vi "Theme4_Topic2_qn8.vi"(9 "RefPrevious":refnum<vi>, 10 "RefNext":refnum<vi>, 11 "connection reference":T1) -> (2 "AnsIndicator":refnum<vi>[](array[refnum]))   [LabVIEW 2013]
uses:
  why.vi
  Precontrol.vi
  <vilib>/addons/database/Connection.llb/Conn ObjectReference.ctl
  <vilib>/addons/database/NI_Database_API.lvlib
panel:
  out "Why?":string
  out "DInd":bool
  out "CInd":bool
  out "BInd":bool
  out "AInd":bool
  in  "ABCD":enum32{"No Selection", "A", "B", "C", "D"}(radio)
  out "MCQ_Randomized":string[](array[string])
  # "The speed of a wave is affected by _____________________."
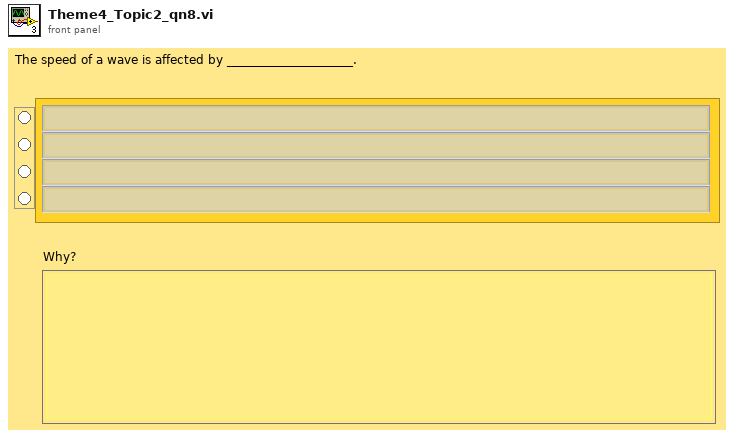
[diagram p1: front panel]
types:
  T1 = typedef "NI_Database_API.lvlib/Conn ObjectReference.ctl" = refnum<k1>
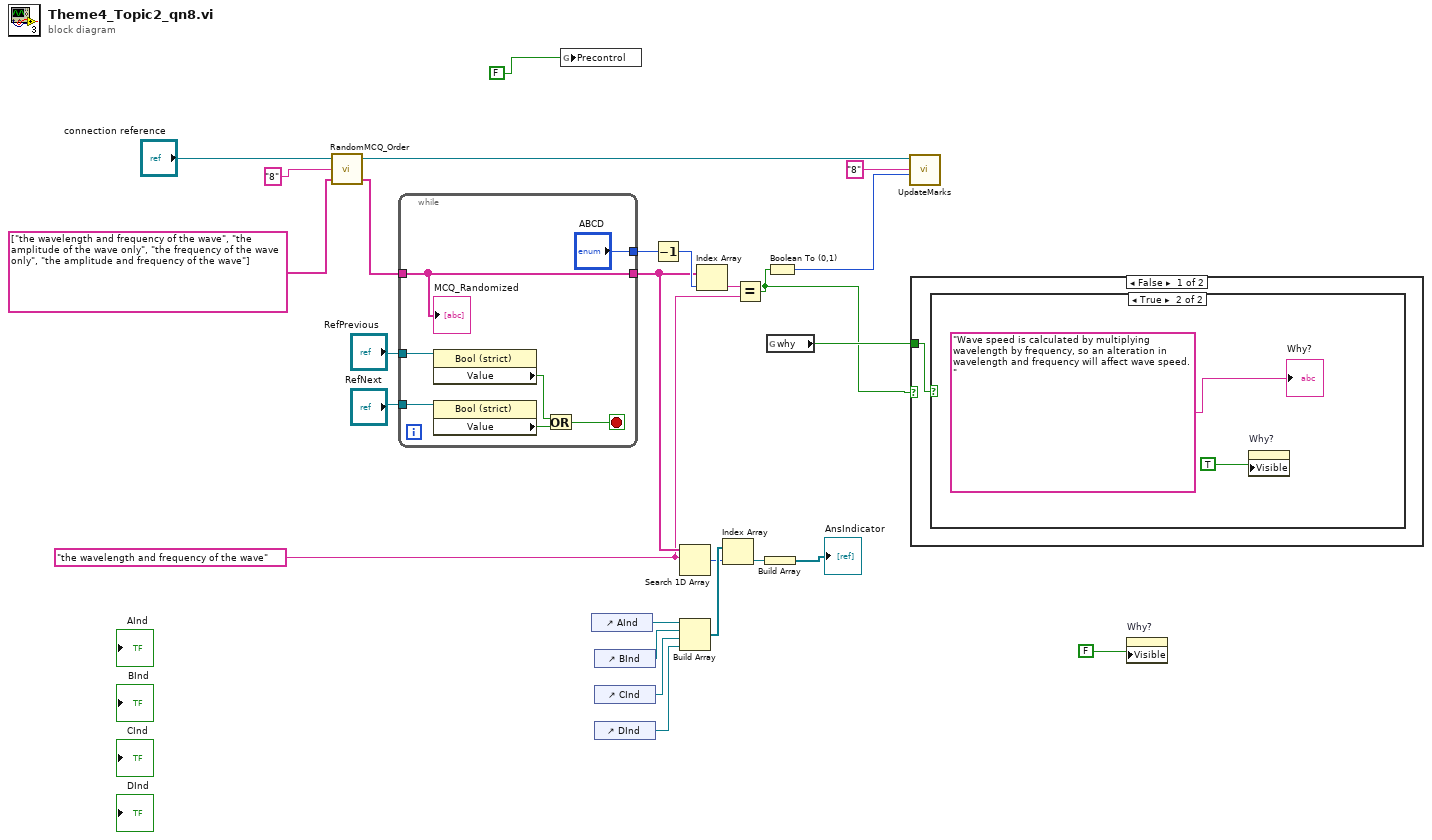
[diagram p0: block diagram]
diagram:
  w13 = "the wavelength and frequency of the wave" ("element")
  n1 = call "RandomMCQ_Order.vi"("MCQ_Ordered"=string[] ["the wavelength and frequency of the wave", "the amplitude of the wave only", "the frequency of the wave only", "the amplitude and frequency of the wave"], "Questions_Ordered"="8", "connection reference"="connection reference") -> ("MCQ_Randomized"=w26:string[], "connection reference out"=w10:T1)  [unwired: 1 in]
  n2 = while {
    tunnel: ["ABCD"] -> w2
    tunnel: w26 -> [w28]
    tunnel: [w28] -> w15
    tunnel: "RefNext" -> [w29]
    tunnel: "RefPrevious" -> [w30]
    stop <- w27 stop-if-true
    n3 = property class="Bool (strict)"(reference=w30) -> ("Value"=w32:bool)  [unwired: 1 in, 2 out]
    n4 = property class="Bool (strict)"(reference=w29) -> ("Value"=w31:bool)  [unwired: 1 in, 2 out]
    n5 = Or(x=w32, y=w31) -> (x .or. y?=w27:bool)
    "MCQ_Randomized" <- w28
  }
  n6 = global write "Precontrol.vi" "Precontrol"(FALSE) -> ()
  n7 = control-ref of="AInd"() -> (w23:refnum<vi>)
  n8 = control-ref of="BInd"() -> (w22:refnum<vi>)
  n9 = control-ref of="CInd"() -> (w21:refnum<vi>)
  n10 = control-ref of="DInd"() -> (w20:refnum<vi>)
  n11 = Decrement(x=w2) -> (x-1=w16:enum32{"No Selection", "A", "B", "C", "D"})
  n12 = Search 1D Array(1D array=w15, element=w13) -> (index of element=w18:i32)  [unwired: 1 in]
  n13 = Build Array(w23, w22, w21, w20) -> (w19:refnum<vi>[])
  n14 = Index Array(array=w15, index=w16) -> (element=w14:string)
  n15 = Index Array(array=w19, index=w18) -> (element=w17:refnum<vi>)
  n16 = Equal?(x=w14, y=w13) -> (x = y?=w4:bool)
  n17 = Build Array(w17) -> (→"AnsIndicator":refnum<vi>[])
  n18 = Boolean To (0,1)(Boolean=w4) -> (0, 1=w6:i16)
  n19 = global read "why.vi" "why"() -> (w5:bool)
  n20 = call "UpdateMarks.vi"("MarksEarned"=w6, "QuestionsNo_Ordered"="8", "connection reference"=w10) -> ()  [unwired: 9 in]
  n21 = case shown="False" w4 {
    tunnel: w5 -> [w34 _]
    frame False {
      n22 = case shown="True" w34 {
        frame False {
        }
        frame True {
          n23 = property on="Why?" class="Str"("Visible"=TRUE) -> ()  [unwired: 2 in, 2 out]
          "Why?" <- "Wave speed is calculated by multiplying wavelength by frequency, so an alteration in wavelength and frequency will affect wave speed."
        }
      }
    }
    frame True {
    }
  }
  n24 = property on="Why?" class="Str"("Visible"=FALSE) -> ()  [unwired: 2 in, 2 out]
